vi "Open Form.vi"(8 "error in (no error)":errorcluster, 10 "Form path":path, 11 "Form Model in":refnum<class "Form Model.lvclass">) -> (0 "error out":errorcluster, 3 "Form Model out":refnum<class "Form Model.lvclass">)   [LabVIEW 2020, in "Form Model.lvlib" / "Form Model.lvclass"]
uses:
  Form Model.lvclass
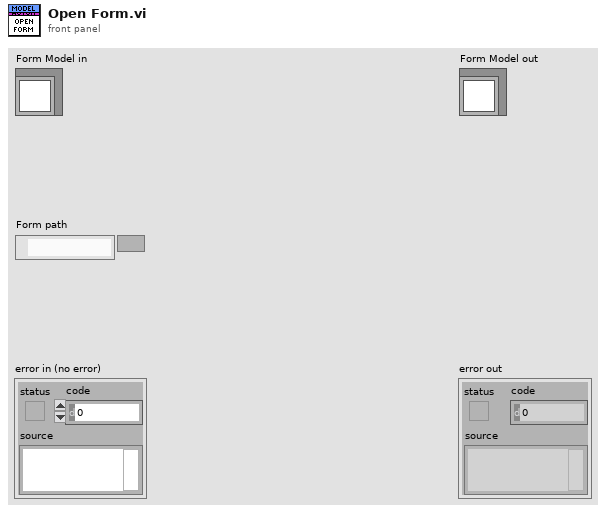
[diagram p1: front panel]
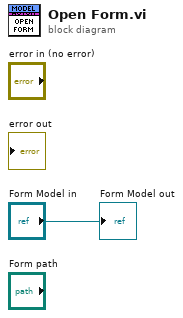
[diagram p0: block diagram]
diagram:
  "Form Model out" <- "Form Model in"
